vi "Call Commands.vi"(10 "Iterations":i32, 11 "Commands":cluster{"Time (s)":dbl, T1, bool}[](array[cluster])) -> ()   [LabVIEW 2019]
uses:
  Support Code/Single Cmd Info.ctl
  <vilib>/picture/picture.llb/imagedata.ctl
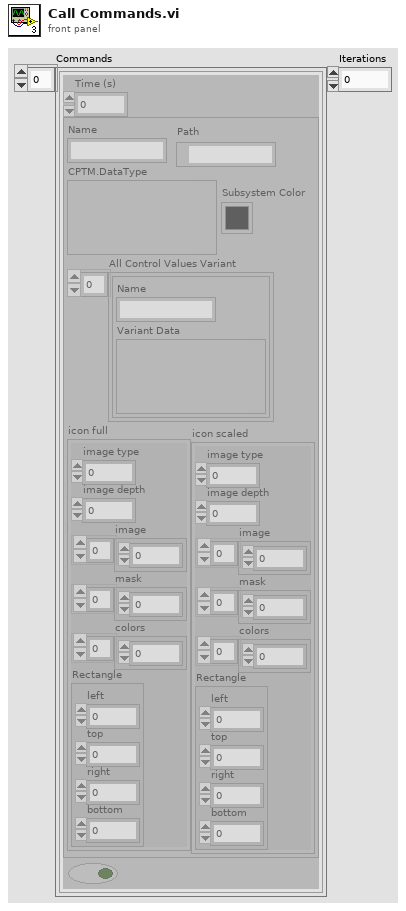
[diagram p1: front panel]
types:
  T1 = typedef "Single Cmd Info.ctl" = cluster{"Name":string, "CPTM.DataType":variant, "All Control Values Variant":cluster{"Name":string, "Variant Data":variant}[], "icon full":T2, "icon scaled":T2, "Path":path, "Subsystem Color":u32}
  T2 = typedef "imagedata.ctl" = cluster{"image type":i32, "image depth":i32, "image":u8[], "mask":u8[], "colors":u32[], "Rectangle":cluster{"left":i16, "top":i16, "right":i16, "bottom":i16}}
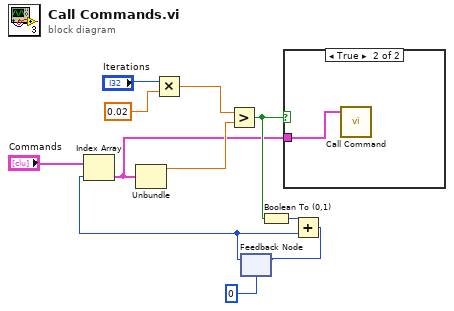
[diagram p0: block diagram]
diagram:
  n1 = Multiply(x="Iterations", y=0.02) -> (x*y=w8:dbl)
  n2 = feedback #1(i16 0) -> (w3:i16)
  n3 = Index Array(array="Commands", index=w3) -> (element=w1:cluster{"Time (s)":dbl, T1, bool})
  n4 = Unbundle(w1) -> ("Time (s)"=w7:dbl)  [unwired: 2 out]
  n5 = Greater?(x=w8, y=w7) -> (0:w6:bool)
  n6 = Boolean To (0,1)(Boolean=w6) -> (0, 1=w5:i16)
  n7 = case shown="True" w6 {
    tunnel: w1 -> [_ w12]
    frame False {
    }
    frame True {
      n8 = call "Call Command.vi"("Command"=w12) -> ()  [unwired: 11 in]
    }
  }
  n9 = Add(x=w5, y=w3) -> (x+y=w4:i16)
  n10 = feedback-in #1(w4) -> ()
